vi "create batch files.vi"(8 "错误输入（无错误）":errorcluster, 9 "Targe Path":path, 10 "Source Path":path, 11 "Batch file":path) -> (0 "错误输出":errorcluster)   [LabVIEW 2016, in "数据传输系统-03.lvlib" / "update.lvlib"]
uses:
  update.lvlib
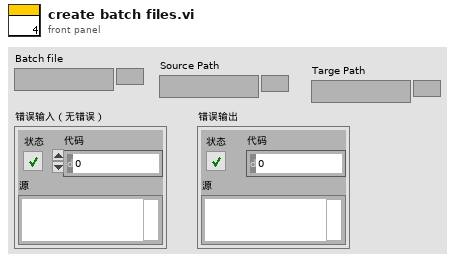
[diagram p1: front panel]
types:
  T1 = enum16{"open", "replace", "create", "open or create", "replace or create", "replace or create with confirmation"}
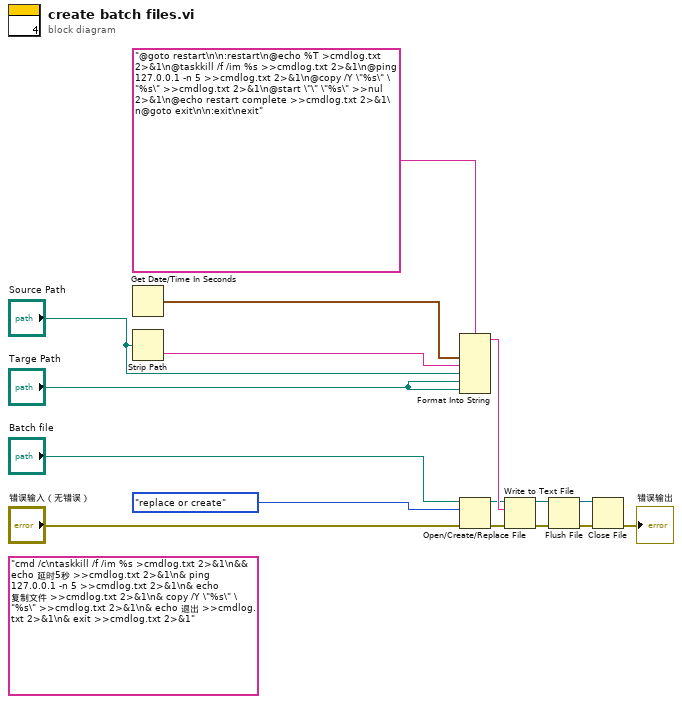
[diagram p0: block diagram]
diagram:
  (unwired) "cmd /c\ntaskkill /f /im %s >cmdlog.txt 2>&1\n&& echo 延时5秒 >>cmdlog.txt 2>&1\n& ping 127.0.0.1 -n 5 >>cmdlog.txt 2>&1\n& echo 复制文件 >>cmdlog.txt 2>&1\n& copy /Y \"%s\" \"%s\" >>cmdlog.txt 2>&1\n& echo 退出 >>cmdlog.txt 2>&1\n& exit >>cmdlog.txt 2>&1" ("名称或相对路径")
  n1 = Get Date/Time In Seconds() -> (seconds since 1Jan1904=w8:timestamp)
  n2 = Strip Path(path="Source Path") -> (name=w14:string)  [unwired: 1 out]
  n3 = Format Into String(format string="@goto restart\n\n:restart\n@echo %T >cmdlog.txt 2>&1\n@taskkill /f /im %s >>cmdlog.txt 2>&1\n@ping 127.0.0.1 -n 5 >>cmdlog.txt 2>&1\n@copy /Y \"%s\" \"%s\" >>cmdlog.txt 2>&1\n@start \"\" \"%s\" >>nul 2>&1\n@echo restart complete >>cmdlog.txt 2>&1\n@goto exit\n\n:exit\nexit" ("文本"), w8, w14, "Source Path", "Targe Path", "Targe Path") -> (resulting string=w11:string)  [unwired: 2 in, 1 out]
  n4 = Open/Create/Replace File(file path (use dialog)="Batch file", error in="错误输入（无错误）", operation (0:open)=T1."replace or create" ("操作(0:open)")) -> (refnum out=w1:refnum<file>, error out=w6:errorcluster)  [unwired: 3 in, 1 out]
  n5 = Write to Text File(file (use dialog)=w1, text=w11, error in=w6) -> (refnum out=w2:refnum<file>, error out=w4:errorcluster)  [unwired: 1 in, 1 out]
  n6 = Flush File(refnum=w2, error in=w4) -> (refnum out=w3:refnum<file>, error out=w5:errorcluster)
  n7 = Close File(refnum=w3, error in=w5) -> (error out=→"错误输出":errorcluster)  [unwired: 1 out]
